vi "KundtsTube.vi"() -> ()   [LabVIEW 2015]
uses:
  <vilib>/imath/engines/lvmath2/RunTimeEngine/Managers/WorkSpace/UID Generator.vi
  <vilib>/imath/engines/lvmath2/RunTimeEngine/RunTimeType/NIMS_RunTimeType_From StrictType (excl LVString).vi
  <instcachedir>/0/NIMS_RunTimeType_From StrictType (excl LVString)_EB1C38A9BC5048DA9ABDA8F781E54D21.lvgen/NIMS_RunTimeType_From StrictType (excl LVString)_EB1C38A9BC5048DA9ABDA8F781E54D21_000.vi
  <vilib>/imath/engines/lvmath2/RunTimeEngine/LocalVariableDefStatement/MC_LocalVariableDefStatement_Display.vi
  <vilib>/imath/engines/lvmath2/RunTimeEngine/Managers/SymbolTable/Clear UID.vi
  <vilib>/imath/engines/lvmath2/RunTimeEngine/NodeEndStatement/NIMS_NodeEndStatement_Output.vi
  <instcachedir>/0/NIMS_NodeEndStatement_Output_53EC0D466D134D7ABD903AC30B43404B.lvgen/NIMS_NodeEndStatement_Output_53EC0D466D134D7ABD903AC30B43404B_009.vi
  <vilib>/imath/engines/lvmath2/RunTimeEngine/ErrorHandling/NIMS_Finalize Error.vi
  <vilib>/Utility/file.llb/Write Delimited Spreadsheet (DBL).vi
  <vilib>/imath/engines/lvmath2/RunTimeEngine/Managers/SymbolTable/NIMS_WorkSpace.lvlib
panel:
  out "RMS (V)":dbl=5.186413371909859
  in  "# of  Samples":dbl=100000.0
  out "Gain vs. Frequency":cluster{i32[], dbl[]}(graph)
  out "Output Freq (Hz)":dbl=10.0
  in  "Sampling Rate (Hz)":dbl=100000.0
  out "Waveform":dynamicdata(graph)=[{"t0"=timestamp(3530658888.3340263 s since 1904-01-01), "dt"=9.999999999999972e-06, "Y"=array[100000 elements], "attributes"=variant("NI_ChannelName"=variant(string "Voltage"), "NI_UnitDescription"=variant(string "Volts"))}]
  in  "Tab Control":enum32{"Sweep", "Single"}(tab)=enum."Single"
  in  "Dwell Time (sec)":dbl=0.5
  in  "Single  Freq (Hz)":i32=10
  in  "Amplitude":dbl=2.0
  in  "freqGen":T1={"Minimum"=10, "Maximum"=10000, "# of Steps"=100, "Spacing"=enum."Linear"}
  in  "Stop Button":bool
  # "This will sweep from min to max, \npausing  by the dwell time  after \neach increment."
  # "Single frequency generation."
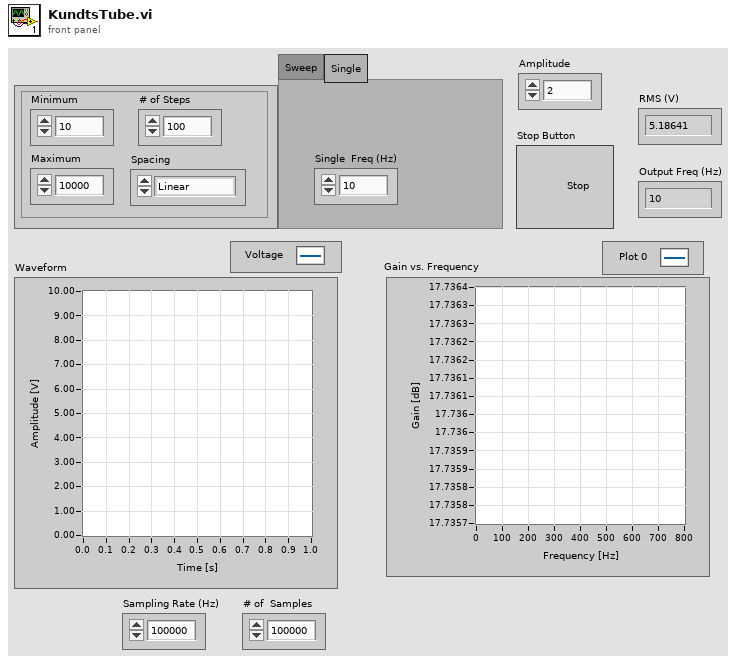
[diagram p1: front panel]
types:
  T1 = cluster{"Minimum":i32, "Maximum":i32, "# of Steps":i32, "Spacing":enum16{"Linear", "Logarithmic"}}
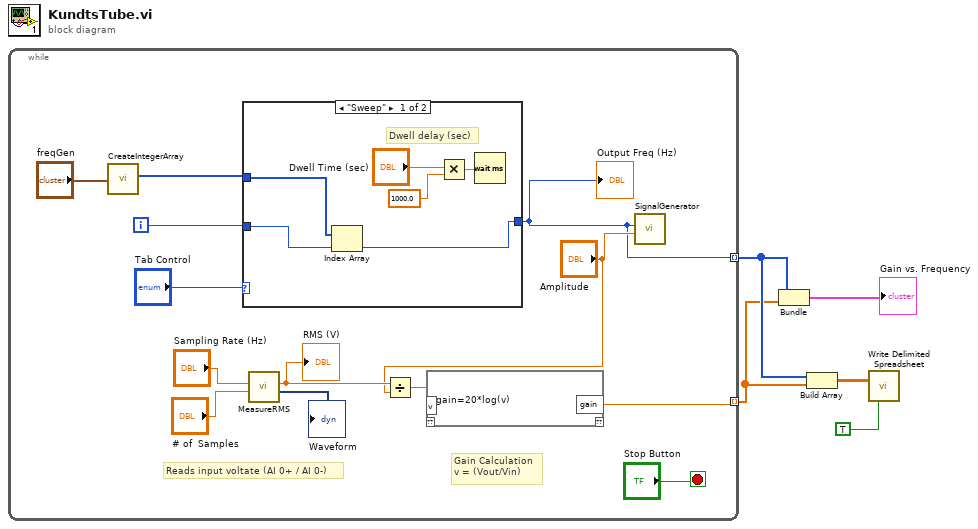
[diagram p0: block diagram]
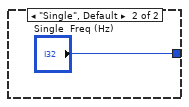
[diagram p2: hidden frame]
diagram:
  n1 = while {
    tunnel: [w6] -> w4 mode=indexing
    tunnel: [w9] -> w2 mode=indexing
    i -> [w11]
    stop <- "Stop Button" stop-if-true
    # "Reads input voltate (AI 0+ / AI 0-)"
    # "Gain Calculation\nv = (Vout/Vin)"
    n2 = call "CreateIntegerArray.vi"("Input Parameters"="freqGen") -> ("Output Array"=w16:i32[])  [unwired: 10 in]
    n3 = case shown="\"Sweep\"" "Tab Control" {
      tunnel: [w56 "Single  Freq (Hz)"] -> w6
      tunnel: w16 -> [w61 _]
      tunnel: w11 -> [w60 _]
      frame "Sweep" {
        # "Dwell delay (sec)"
        n4 = Index Array "Index Array"(array=w61, index=w60) -> (element=w56:i32)
        n5 = Multiply(x="Dwell Time (sec)", y=1000.0 ("x")) -> (x*y=w59:dbl)
        n6 = Wait (ms)(milliseconds to wait=w59) -> ()  [unwired: 1 out]
      }
      frame "Single", Default {
      }
    }
    "Output Freq (Hz)" <- w6
    n7 = call "MeasureRMS.vi"("Samples"="# of  Samples", "Sampling Rate"="Sampling Rate (Hz)") -> ("Waveform Graph"=→"Waveform":dynamicdata, "RMS"=w13:dbl)  [unwired: 6 in, 1 out]
    "RMS (V)" <- w13
    n8 = Divide(x=w13, y="Amplitude") -> (x/y=w10:dbl)
    n9 = mathscript code="gain=20*log(v)"("v"=w10) -> ("gain"=w9:cdb)  [unwired: 1 in, 1 out]
    n10 = call "SignalGenerator.vi"("Frequency"=w6, "Amplitude"="Amplitude") -> ()  [unwired: 8 in, 1 out]
  }
  n11 = Bundle(w4, w2) -> (→"Gain vs. Frequency":cluster{i32[], cdb[]})  [unwired: 1 in]
  n12 = Build Array(w4, w2) -> (w3:cdb[][])
  n13 = call-poly <vilib>:"Write Delimited Spreadsheet.vi"("2D data"=w3, "transpose? (F)"=TRUE) -> ()  [unwired: 12 in, 2 out]
